vi "Master_ActuatorStates.vi"(8 "error in (no error)":errorcluster) -> (0 "error out":errorcluster, 2 "CurrentActuations":T1={"Pod Power"=FALSE, "Release Valve"=TRUE, "Brakes"=FALSE, "Clamp"=FALSE, "Ignition"=FALSE, "Pump"=FALSE, "Motor Forward"=FALSE, "Motor Reverse"=FALSE})   [LabVIEW 2017]
doc: "Reads state of actuators and formats it for data stream."
uses:
  Control/TypeDef_DigitalOuts.ctl
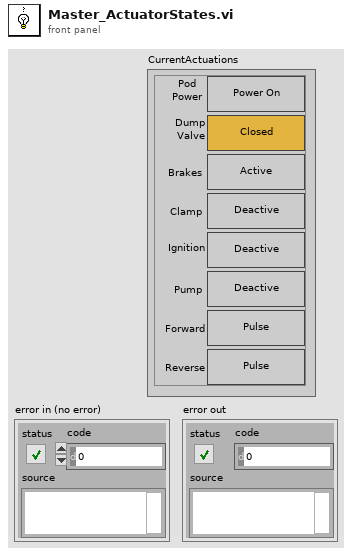
[diagram p1: front panel]
types:
  T1 = typedef "TypeDef_DigitalOuts.ctl" = cluster{"Pod Power":bool, "Release Valve":bool, "Brakes":bool, "Clamp":bool, "Ignition":bool, "Pump":bool, "Motor Forward":bool, "Motor Reverse":bool}
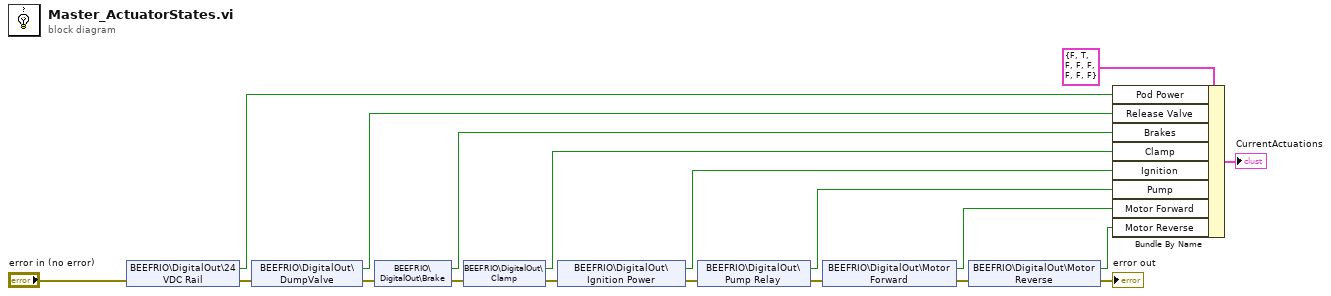
[diagram p0: block diagram]
diagram:
  n1 = shared-variable "BEEFRIO\\DigitalOut\\24 VDC Rail"(error in="error in (no error)") -> (w8:bool, error out=w19:errorcluster)
  n2 = shared-variable "BEEFRIO\\DigitalOut\\DumpValve"(error in=w19) -> (w7:bool, error out=w18:errorcluster)
  n3 = shared-variable "BEEFRIO\\DigitalOut\\Brake"(error in=w18) -> (w6:bool, error out=w17:errorcluster)
  n4 = shared-variable "BEEFRIO\\DigitalOut\\Clamp"(error in=w17) -> (w5:bool, error out=w13:errorcluster)
  n5 = shared-variable "BEEFRIO\\DigitalOut\\Ignition Power"(error in=w13) -> (w4:bool, error out=w16:errorcluster)
  n6 = shared-variable "BEEFRIO\\DigitalOut\\Pump Relay"(error in=w16) -> (w3:bool, error out=w15:errorcluster)
  n7 = shared-variable "BEEFRIO\\DigitalOut\\Motor Forward"(error in=w15) -> (w2:bool, error out=w14:errorcluster)
  n8 = shared-variable "BEEFRIO\\DigitalOut\\Motor Reverse"(error in=w14) -> (w1:bool, error out=→"error out":errorcluster)
  n9 = Bundle By Name(cluster=T1 {"Pod Power"=FALSE, "Release Valve"=TRUE, "Brakes"=FALSE, "Clamp"=FALSE, "Ignition"=FALSE, "Pump"=FALSE, "Motor Forward"=FALSE, "Motor Reverse"=FALSE} ("Actuators"), "Pod Power"=w8, "Release Valve"=w7, "Brakes"=w6, "Clamp"=w5, "Ignition"=w4, "Pump"=w3, "Motor Forward"=w2, "Motor Reverse"=w1) -> (→"CurrentActuations":T1)
